vi "lockin.GetEvents.vi"(8 "error in (no error)":errorcluster, 11 "system in":refnum<class "system.lvclass">) -> (0 "error out":errorcluster, 3 "Event Registration Refnum":refnum<event-registration>)   [LabVIEW 2016, in "system.lvclass"]
uses:
  system.lvclass
  <vilib>/JKI/JKI SMO/SMO/Typedefs/Protected Events.ctl
  <vilib>/JKI/JKI SMO/SMO/Typedefs/StopProcessEventData--Cluster.ctl
  <vilib>/JKI/JKI SMO/SMO/Typedefs/AbortProcessEventData--Cluster.ctl
  <vilib>/JKI/JKI SMO/SMO/Typedefs/SMO Dependency Event--Cluster.ctl
  <vilib>/JKI/JKI SMO/SMO/Typedefs/SMO Dependency Event--Enum.ctl
  Typedefs/PrivateEvents--Cluster.ctl
  Typedefs/PrivateEvents--lockin.output_config.ctl
  Typedefs/PrivateEvents--lockin.runCalculation.ctl
  DSP/Typedefs/LP_Config.ctl
  DSP.lockin/Typedefs/Lockin_Config.ctl
  DSP/Typedefs/FFT_Config.ctl
  <vilib>/Analysis/4window.llb/windowTd.ctl
  <vilib>/measure/maspectr.llb/Power Spectrum and PSD Export Mode.ctl
  Typedefs/PrivateEvents--lockin.lockin_REF_waveform.ctl
  <vilib>/JKI/JKI SMO/SMO/Typedefs/Public Events.ctl
  <vilib>/JKI/JKI SMO/SMO/Typedefs/SMOState --Enum.ctl
  <vilib>/JKI/JKI SMO/SMO/Typedefs/Reserve State--Enum.ctl
  DAQ_Manager/Typedefs/PublicEvents--Cluster.ctl
  DAQ_Manager/Typedefs/PublicEvents--DAQ_Manager.getWaveform.ctl
  DSP/Typedefs/PublicEvents--Cluster.ctl
  DSP/Typedefs/PublicEvents--DSP.getWaveforms.ctl
  DSP/Typedefs/PublicEvents--DSP.getLockin.ctl
  DSP.lockin/Typedefs/LockinResult.ctl
  DSP/Typedefs/PublicEvents--DSP.getPowerSpectrum.ctl
  Generator/Typedefs/PublicEvents--Cluster.ctl
  Generator/Typedefs/PublicEvents--Generator.getGeneratorWaveforms.ctl
  system.lvclass/system.ctl
  DAQ_Manager/DAQ_Manager.lvclass
  DSP/DSP.lvclass
  Generator/Generator.lvclass
  <vilib>/JKI/JKI SMO/SMO/SMO.lvclass
  DSP.lockin/DSP_lockin.lvclass
  <vilib>/Analysis/NI_AALPro.lvlib
  <vilib>/measure/NI_MAPro.lvlib
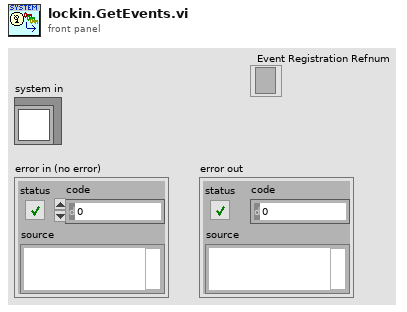
[diagram p1: front panel]
types:
  T1 = typedef "SMO.lvclass/Protected Events.ctl" = cluster{"StopProcesses":refnum<user-event>, "AbortProcesses":refnum<user-event>, "Config Changed":refnum<user-event>, "Dependency":refnum<user-event>}
  T2 = typedef "system.lvclass/PrivateEvents--Cluster.ctl" = cluster{"output_config":refnum<user-event>, "lockin_config":refnum<user-event>, "lockin_REF_waveform":refnum<user-event>}
  T3 = cluster{"SMO Protected Events":T1, "Private Events":T2}
  T4 = typedef "SMO.lvclass/Public Events.ctl" = cluster{"Error":refnum<user-event>, "State":refnum<user-event>, "Reserve State":refnum<user-event>}
  T5 = typedef "DAQ_Manager.lvclass/PublicEvents--Cluster.ctl" = cluster{"getWaveform":refnum<user-event>}
  T6 = typedef "DSP.lvclass/PublicEvents--Cluster.ctl" = cluster{"getWaveforms":refnum<user-event>, "getLockin":refnum<user-event>, "getPowerSpectrum":refnum<user-event>}
  T7 = typedef "Generator.lvclass/PublicEvents--Cluster.ctl" = cluster{"getGeneratorWaveforms":refnum<user-event>}
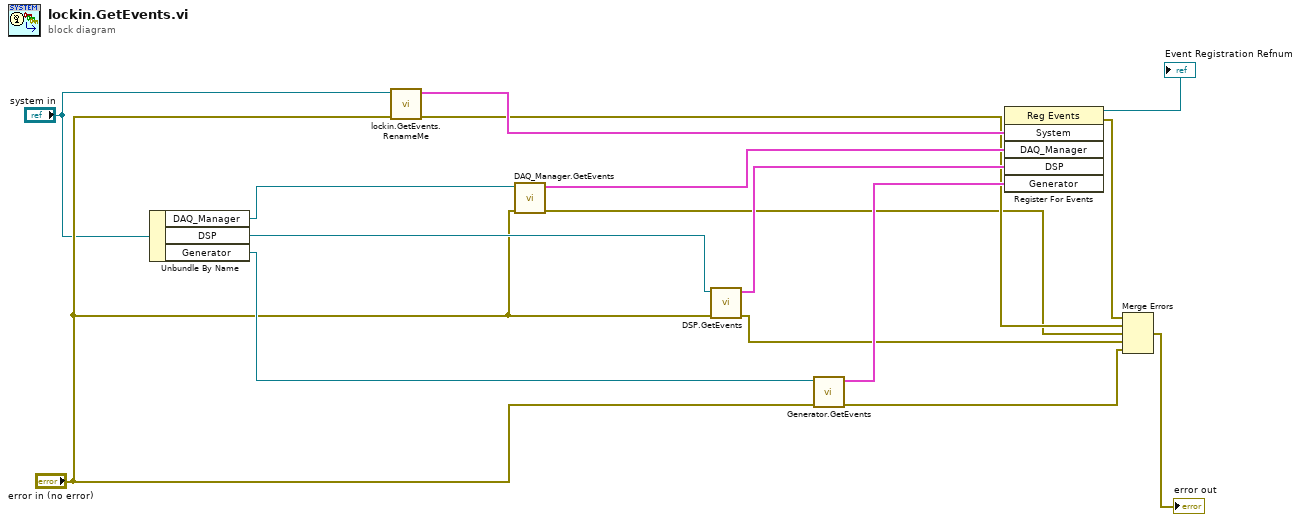
[diagram p0: block diagram]
diagram:
  n1 = Unbundle By Name("system in") -> ("DAQ_Manager"=w14:refnum<class "DAQ_Manager.lvclass">, "DSP"=w11:refnum<class "DSP.lvclass">, "Generator"=w12:refnum<class "Generator.lvclass">)
  n2 = call "lockin.GetEvents.RenameMe.vi"("error in (no error)"="error in (no error)", "system in"="system in") -> ("error out"=w3:errorcluster, "System"=w10:T3)  [unwired: 8 in]
  n3 = call "DAQ_Manager.GetEvents.vi"("error in (no error)"="error in (no error)", "DAQ_Manager in"=w14) -> ("error out"=w2:errorcluster, "DAQ_Manager"=w9:cluster{"Public Events":T4, "Public Events":T5})  [unwired: 8 in]
  n4 = call "DSP.GetEvents.vi"("error in (no error)"="error in (no error)", "DSP in"=w11) -> ("error out"=w1:errorcluster, "DSP"=w8:cluster{"Public Events":T4, "Public Events":T6})  [unwired: 8 in]
  n5 = call "Generator.GetEvents.vi"("error in (no error)"="error in (no error)", "Generator in"=w12) -> ("error out"=w6:errorcluster, "Generator"=w7:cluster{"Public Events":T4, "Public Events":T7})  [unwired: 8 in]
  n6 = register-events(w10, w9, w8, w7) -> (reference out=→"Event Registration Refnum":refnum<event-registration>, error out=w16:errorcluster)  [unwired: 2 in]
  n7 = Merge Errors(w16, w3, w2, w1, w6) -> (→"error out":errorcluster)
